vi "GetChirp.vi"(8 "error in (no error)":errorcluster, 11 "reference in":refnum<class "metadata.lvclass">) -> (0 "error out":errorcluster, 2 "Chirp":T1, 3 "reference out":refnum<class "metadata.lvclass">)   [LabVIEW 2019, in "metadata.lvclass"]
uses:
  metadata.lvclass
  Chirp added parameters.ctl
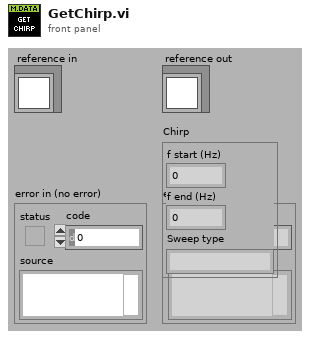
[diagram p1: front panel]
types:
  T1 = typedef "metadata.lvclass/Chirp added parameters.ctl" = cluster{"f start (Hz)":dbl, "f end (Hz)":dbl, "Sweep type":string}
  T2 = typedef "metadata.lvclass/ObjectAttributesRef.ctl" = refnum<data-value>
  T3 = typedef "metadata.lvclass/ObjectAttributes.ctl" = cluster{"MyAttribute":dbl, "System Control":T4, "file info":T5, "Sample info":T6, "Cantilever info":T7, "XYZ piezos":T8, "Mapping":T9, "Fcurve segment":T10[], "Fast fpga segment":T12, "Chirp":T1, "precision (6)":i16, "width (-)":i16, "Metadata":T13, "config filepath":path, "Section names []":string[], "Property names []":string[], "nb elements":u16}
  T4 = typedef "metadata.lvclass/System control parameters.ctl" = cluster{"FPGA SW version":string, "TDMS file version":string, "Instrument":string, "Instrument model":string, "Instrument scanner":string, "Instrument clockrate (Mhz)":string, "Instrument tick time (us)":string}
  T5 = typedef "metadata.lvclass/File info parameters.ctl" = cluster{"Time Stamp":timestamp, "Filename":string, "Filepath":path, "User":string, "Experiment_name":string, "Curve_id":string, "number_segments":u8, "number_consecutive_scans":u32}
  T6 = typedef "metadata.lvclass/Sample info parameters.ctl" = cluster{"Sample name":string, "Sample species":string}
  T7 = typedef "metadata.lvclass/Cantilever info parameters.ctl" = cluster{"spring constant calib method":string, "invOLS calib method":string, "thermal calib deflection channel":string, "model":string, "shape":string, "tip geometry":string, "Laser sum (V)":dbl, "Laser power (mA)":dbl, "invOLS_(nm/V)":dbl, "spring constant nominal (N/m)":dbl, "spring constant calib (N/m)":dbl, "resosnance frequency air calib (Hz)":dbl, "resosnance frequency calib (Hz)":dbl, "quality factor":dbl, "Acoefficident_GCI_(nN.s^1.3/m)":dbl, "half angle (deg)":dbl, "tip radius (m)":dbl, "tip height (m)":dbl, "system mount angle (deg)":dbl}
  T8 = typedef "metadata.lvclass/XYZ piezos parameters.ctl" = cluster{"X stage piezo sensitivity (nm/V)":dbl, "X stage piezo gain":dbl, "X velocity (V/tick)":dbl, "X closed loop":bool, "Y stage piezo sensitivity (nm/V)":dbl, "Y stage piezo gain":dbl, "Y velocity (V/tick)":dbl, "Y closed loop":bool, "Z stage piezo sensitivity (nm/V)":dbl, "Z stage piezo gain":dbl, "Z closed loop":bool, "X position (V)":dbl, "Y position (V)":dbl}
  T9 = typedef "metadata.lvclass/Mapping parameters.ctl" = cluster{"Mapping":bool, "index":u16, "position row":u16, "position column":u16, "next position row":i16, "next position column":i16, "X initial position (V)":dbl, "Y initial position (V)":dbl, "X step size (V)":dbl, "Y step size (V)":dbl}
  T10 = typedef "metadata.lvclass/Fcurve segment.ctl" = cluster{"type":T11, "fast_fpga_trigger":bool, "nb":u8, "duration (ticks)":i64, "nb points":i32, "sampling rate (S/s)":u32, "Zpiezo control out":string, "initial deflection (V)":dbl, "relative setpoint":bool, "setpoint on":bool, "setpoint (V)":dbl, "setpoint trigger channel":string, "velocity (V/tick)":dbl, "Z position setpoint trigger (V)":dbl, "Z retract length (V)":dbl, "dec factor":u32}
  T11 = typedef "metadata.lvclass/Segment type--combobox.ctl" = string
  T12 = typedef "metadata.lvclass/fast fpga segment parameters.ctl" = cluster{"Fast start time trigger":timestamp, "nb_points":u32, "sampling_rate_(S/s)":u32, "duration_(ticks)":u32}
  T13 = typedef "metadata.lvclass/Metadata output --cluster.ctl" = cluster{"Property Names":string[], "Property Values":variant[]}
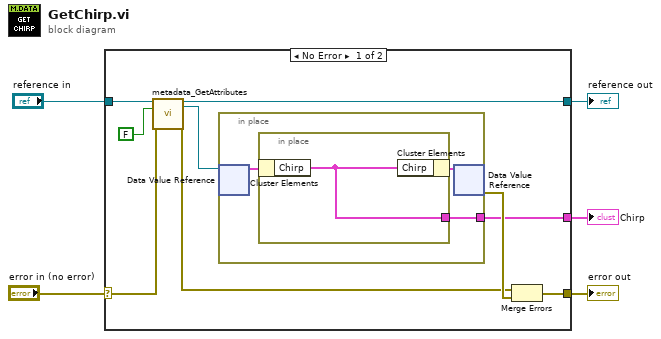
[diagram p0: block diagram]
diagram:
  n1 = case shown="No Error" "error in (no error)" {
    selector: "error in (no error)" -> [w14 w20]
    tunnel: [w8 w20] -> w4
    tunnel: [w13 w19] -> w2
    tunnel: "reference in" -> [w12 w19]
    tunnel: [w6 _] -> w1
    frame No Error {
      n2 = call "metadata_GetAttributes.vi"("reference in"=w12, "return data? (T)"=FALSE, "error in (no error)"=w14) -> ("reference out"=w13:refnum<class "metadata.lvclass">, "attributes ref"=w7:T2, "error out"=w9:errorcluster)  [unwired: 13 in, 1 out]
      n3 = in-place {
        in-place-border: [w15] -> w6
        n4 = in-place-dvr #1(w7) -> (w16:T3)  [unwired: 1 out]
        n5 = in-place {
          in-place-border: [w18] -> w15
          n6 = in-place-cluster #2(w16) -> ("Chirp"=w18:T1)
          n7 = in-place-cluster #2("Chirp"=w18) -> (w17:T3)
        }
        n8 = in-place-dvr #1(w17) -> (w10:errorcluster)  [unwired: 1 out]
      }
      n9 = Merge Errors(w9, w10) -> (w8:errorcluster)
    }
    frame Error {
    }
  }
  "error out" <- w4
  "reference out" <- w2
  "Chirp" <- w1
